vi "Menu_Create.vi"(6 "Vegetarian":bool, 7 "Price":dbl, 8 "Error In":errorcluster, 9 "Description":string, 10 "Name":string, 11 "reference in":refnum<class "Menu.lvclass">) -> (0 "Error Out":errorcluster, 3 "reference out":refnum<class "Menu.lvclass">)   [LabVIEW 2020, in "Menu.lvclass"]
uses:
  Menu.lvclass
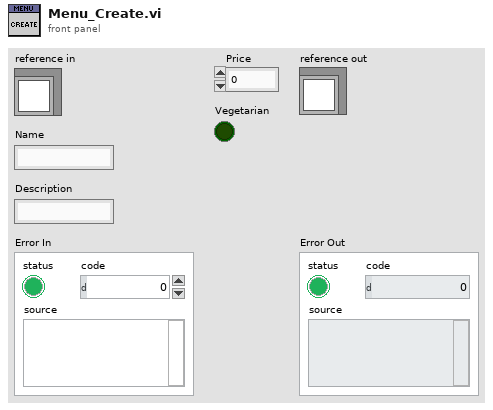
[diagram p1: front panel]
types:
  T1 = typedef "Menu.lvclass/ObjectAttributes.ctl" = cluster{"Name":string, "Description":string, "Vegetarian":bool, "Price":dbl}
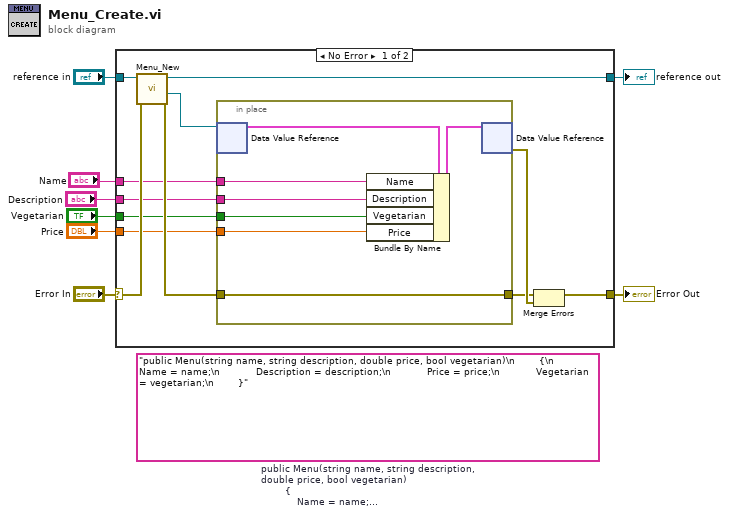
[diagram p0: block diagram]
diagram:
  (unwired) "public Menu(string name, string description, double price, bool vegetarian)\n        {\n            Name = name;\n            Description = description;\n            Price = price;\n            Vegetarian = vegetarian;\n        }"  # public Menu(string name, string description, double price, bool vegetarian)         {             Name = name;             Description = description;             Price = price;             Vegetarian = vegetarian;         }
  n1 = case shown="No Error" "Error In" {
    selector: "Error In" -> [w19 w29]
    tunnel: [w13 w29] -> w7
    tunnel: "reference in" -> [w20 w28]
    tunnel: [w18 w28] -> w5
    tunnel: "Name" -> [w12 _]
    tunnel: "Description" -> [w11 _]
    tunnel: "Price" -> [w10 _]
    tunnel: "Vegetarian" -> [w9 _]
    frame No Error {
      n2 = call "Menu_New.vi"("error in (no error)"=w19, "reference in"=w20) -> ("error out"=w15:errorcluster, "DVRRefOut"=w16:refnum<data-value>, "reference out"=w18:refnum<class "Menu.lvclass">)  [unwired: 6 in, 1 out]
      n3 = in-place {
        in-place-border: w15 -> [w25]
        in-place-border: [w25] -> w14
        in-place-border: w12 -> [w24]
        in-place-border: w11 -> [w23]
        in-place-border: w10 -> [w22]
        in-place-border: w9 -> [w21]
        n4 = in-place-dvr #1(w16) -> (w26:T1)  [unwired: 1 out]
        n5 = Bundle By Name(cluster=w26, "Name"=w24, "Description"=w23, "Vegetarian"=w21, "Price"=w22) -> (w27:T1)
        n6 = in-place-dvr #1(w27) -> (w17:errorcluster)  [unwired: 1 out]
      }
      n7 = Merge Errors(w14, w17) -> (w13:errorcluster)
    }
    frame Error {
      # "VI-TechBaseTemplate_Simple_4x4x4"
    }
  }
  "Error Out" <- w7
  "reference out" <- w5
